vi "Read Voltage (Linear Current Sweep).vi"(5 "Delay Time (0.01 S)":dbl=0.01, 6 "Pulse Stop Level (0.01 A)":dbl=0.01, 7 "Sweep Points (10)":i32=10, 8 "error in (no error)":errorcluster, 9 "Pulse Start Level (-0.01 A)":dbl=-0.01, 10 "Source Measure Unit Channel (0: Channel A)":i32(ring) items=["Channel A", "Channel B"], 11 "VISA resource name":refnum<visa-resource-name>) -> (0 "error out":errorcluster, 2 "Voltage (V)":dbl[](array[numeric]), 3 "VISA resource name out":refnum<visa-resource-name>)   [LabVIEW 2015, in "Keithley 2600 Series.lvlib"]
doc: "Performs a linear current sweep with voltage measured at every point."
uses:
  Keithley 2600 Series.lvlib
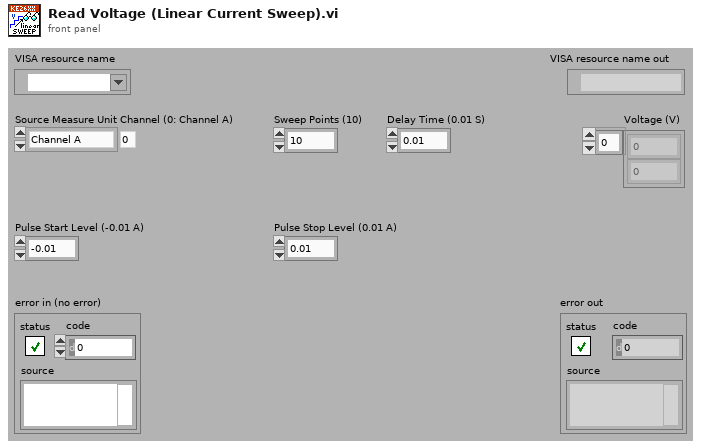
[diagram p1: front panel]
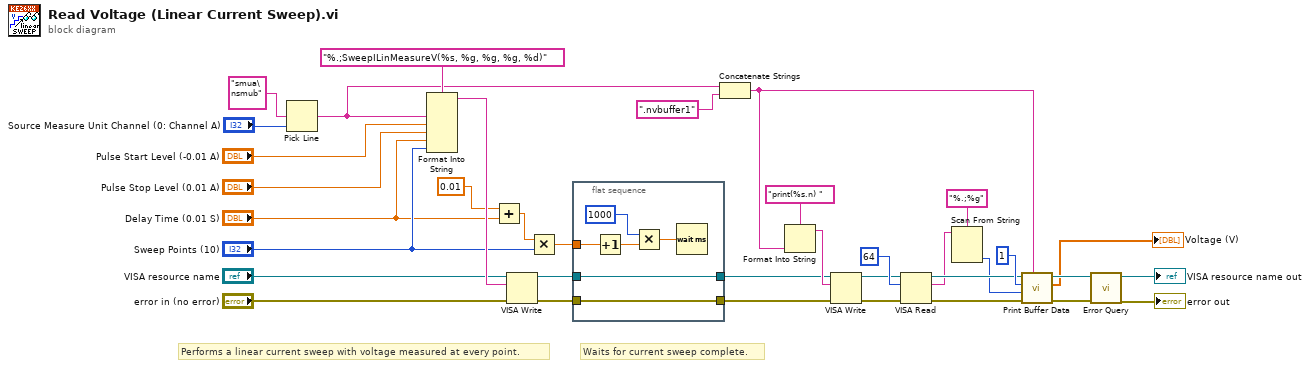
[diagram p0: block diagram]
diagram:
  # "Waits for current sweep complete."
  # "Performs a linear current sweep with voltage measured at every point."
  n1 = Pick Line(multi-line string="smua\nsmub", line index="Source Measure Unit Channel (0: Channel A)") -> (output string=w3:string)  [unwired: 1 in]
  n2 = Format Into String(format string="%.;SweepILinMeasureV(%s, %g, %g, %g, %d)", w3, "Pulse Start Level (-0.01 A)", "Pulse Stop Level (0.01 A)", "Delay Time (0.01 S)", "Sweep Points (10)") -> (resulting string=w33:string)  [unwired: 2 in, 1 out]
  n3 = Add(x=0.01, y="Delay Time (0.01 S)") -> (x+y=w22:dbl)
  n4 = VISA Write(VISA resource name="VISA resource name", write buffer=w33, error in (no error)="error in (no error)") -> (VISA resource name out=w26:refnum<visa-resource-name>, error out=w25:errorcluster)  [unwired: 1 out]
  n5 = Multiply(x=w22, y="Sweep Points (10)") -> (x*y=w23:dbl)
  n6 = flat-sequence {
    tunnel: w26 -> [w42]
    tunnel: w25 -> [w41]
    tunnel: [w42] -> w7
    tunnel: [w41] -> w6
    tunnel: w23 -> [w38]
    frame #0 {
      n7 = Increment(x=w38) -> (x+1=w37:dbl)
      n8 = Multiply(x=1000, y=w37) -> (x*y=w39:dbl)
      n9 = Wait (ms)(milliseconds to wait=w39) -> ()  [unwired: 1 out]
    }
  }
  n10 = Concatenate Strings(w3, ".nvbuffer1" ("string")) -> (w2:string)
  n11 = Format Into String(format string="print(%s.n) ", w2) -> (resulting string=w9:string)  [unwired: 2 in, 1 out]
  n12 = VISA Write(VISA resource name=w7, write buffer=w9, error in (no error)=w6) -> (VISA resource name out=w12:refnum<visa-resource-name>, error out=w11:errorcluster)  [unwired: 1 out]
  n13 = VISA Read(VISA resource name=w12, byte count=u32 64, error in (no error)=w11) -> (VISA resource name out=w17:refnum<visa-resource-name>, read buffer=w15:string, error out=w16:errorcluster)  [unwired: 1 out]
  n14 = Scan From String(format string="%.;%g", input string=w15) -> (output 1=w14:i32)  [unwired: 3 in, 3 out]
  n15 = call "Print Buffer Data.vi"("Reading Buffer (smua.nvbuffer1)"=w2, "error in (no error)"=w16, "End Index (1)"=w14, "Start Index (1)"=1 ("Start Index (0)"), "VISA resource name"=w17) -> ("error out"=w4:errorcluster, "Buffer Data"=→"Voltage (V)":dbl[], "VISA resource name out"=w5:refnum<visa-resource-name>)  [unwired: 4 in]
  n16 = call "Error Query.vi"("error in (no error)"=w4, "VISA resource name"=w5) -> ("error out"=→"error out":errorcluster, "VISA resource name out"=→"VISA resource name out":refnum<visa-resource-name>)  [unwired: 6 in, 2 out]
